vi "Write File.vi"(7 "Address":string, 8 "Error In":errorcluster) -> (0 "Error Out":errorcluster)   [LabVIEW 2018, in "Tests.lvlib" / "Known Hosts.lvlib"]
uses:
  Known Hosts.lvlib
  <vilib>/Utility/error.llb/Clear Errors.vi
  <vilib>/Utility/sysdir.llb/Get System Directory.vi
  <vilib>/addons/_JKI Toolkits/Caraya/classes/Test/Test.lvclass
  <vilib>/addons/_JKI Toolkits/Caraya/classes/Assert/Assert.lvclass
  src/Toolkit/Known Hosts/Known Hosts.lvclass
  Tests.lvlib
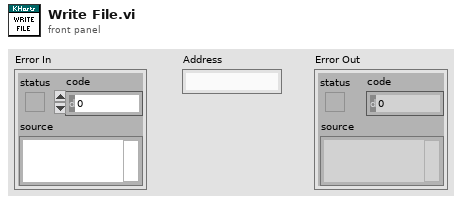
[diagram p1: front panel]
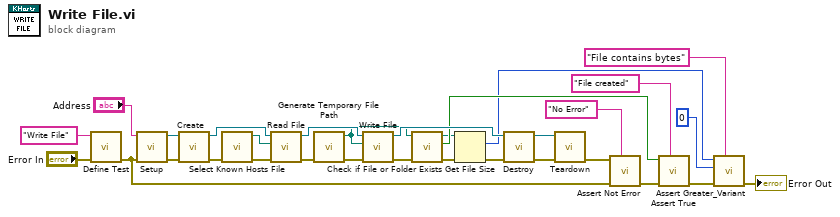
[diagram p0: block diagram]
diagram:
  n1 = call <vilib>:"Define Test.vi"("error in (no error)"="Error In", "Label (VI Title)"="Write File") -> ("error out"=w6:errorcluster)  [unwired: 9 in]
  n2 = call "Setup.vi"("Error In"=w6, "Address In"="Address") -> ("Error Out"=w5:errorcluster, "Sesssion"=w2:refnum<class "Session.lvclass">)  [unwired: 7 in, 1 out]
  n3 = call "Create.vi"("Error In"=w5, "Session"=w2) -> ("Error Out"=w27:errorcluster, "Known Hosts"=w28:refnum<class "Known Hosts.lvclass">)  [unwired: 8 in]
  n4 = call "Select Known Hosts File.vi"("Error In"=w27) -> ("Error Out"=w26:errorcluster, "Known Hosts File"=w25:path)  [unwired: 9 in]
  n5 = call "Read File.vi"("Error In"=w26, "File"=w25, "KnownHosts In"=w28) -> ("Error Out"=w22:errorcluster, "KnownHosts Out"=w24:refnum<class "Known Hosts.lvclass">)  [unwired: 6 in, 1 out]
  n6 = call <vilib>:"Generate Temporary File Path.vi"("error in (no error)"=w22) -> ("error out"=w21:errorcluster, "Unique Temporary File Path"=w19:path)  [unwired: 9 in]
  n7 = call "Write File.vi"("Error In"=w21, "File"=w19, "KnownHosts In"=w24) -> ("Error Out"=w20:errorcluster, "KnownHosts Out"=w23:refnum<class "Known Hosts.lvclass">)  [unwired: 7 in]
  n8 = call <vilib>:"Check if File or Folder Exists.vi"("error in (no error)"=w20, "path"=w19) -> ("error out"=w13:errorcluster, "file or folder exists?"=w18:bool, "dup path"=w14:path)  [unwired: 7 in]
  n9 = Get File Size(file=w14, error in=w13) -> (size (in bytes)=w9:i64, 0:w12:errorcluster)  [unwired: 1 out]
  n10 = call "Destroy.vi"("Error In"=w12, "KnownHosts"=w23) -> ("Error Out"=w4:errorcluster, "Session"=w1:refnum<class "Session.lvclass">)  [unwired: 8 in]
  n11 = call "Teardown.vi"("Error In"=w4, "Session"=w1) -> ("Error Out"=w3:errorcluster)  [unwired: 9 in]
  n12 = call <vilib>:"Assert Not Error.vi"("Label"="No Error", "error in (no error)"=w6, "Not Error?"=w3) -> ("error out"=w17:errorcluster)  [unwired: 8 in]
  n13 = call <vilib>:"Assert True.vi"("Label"="File created", "error in (no error)"=w17, "True?"=w18) -> ("error out"=w16:errorcluster)  [unwired: 8 in]
  n14 = call <vilib>:"Assert Greater_Variant.vi"("Label"="File contains bytes", "error in (no error)"=w16, "Y"=i64 0 ("size (in bytes)"), "X"=w9) -> ("error out"=→"Error Out":errorcluster)  [unwired: 7 in]
